vi "Write Editable From.vi"(8 "error in (no error)":errorcluster, 10 "RowAndCollumn":T1, 11 "MCListbox View in":refnum<class "MCListbox View.lvclass">) -> (0 "error out":errorcluster, 3 "MCListbox View out":refnum<class "MCListbox View.lvclass">)   [LabVIEW 2013, in "SET Project Editor.lvlib" / "MCListbox View.lvclass"]
uses:
  MCListbox View.lvclass
  <vilib>/Utility/miscctls.llb/LVRowAndColumnTypeDef.ctl
  MCListbox View.lvclass/MCListbox View.ctl
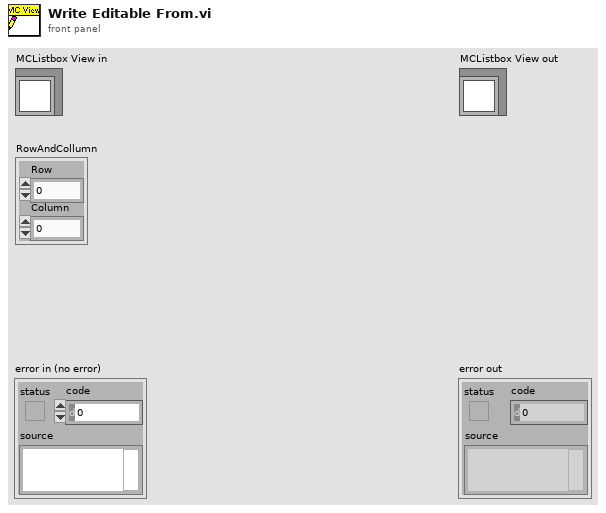
[diagram p1: front panel]
types:
  T1 = typedef "LVRowAndColumnTypeDef.ctl" = cluster{"Row":i32, "Column":i32}
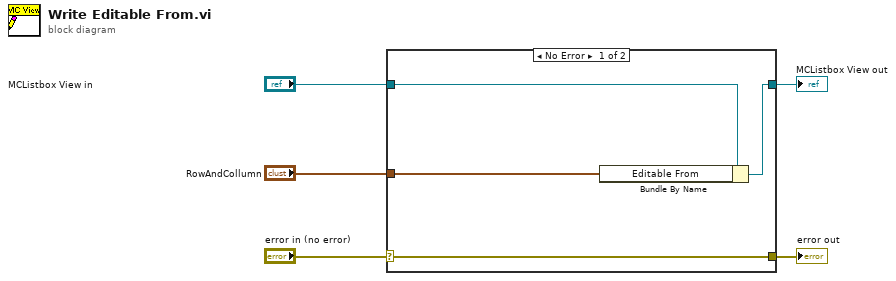
[diagram p0: block diagram]
diagram:
  n1 = case shown="No Error" "error in (no error)" {
    selector: "error in (no error)" -> [w9 w10]
    tunnel: [w9 w10] -> w4
    tunnel: [w7 w11] -> w2
    tunnel: "MCListbox View in" -> [w8 w11]
    tunnel: "RowAndCollumn" -> [w6 _]
    frame No Error {
      n2 = Bundle By Name(cluster=w8, "Editable From"=w6) -> (w7:refnum<class "MCListbox View.lvclass">)
    }
    frame Error {
    }
  }
  "error out" <- w4
  "MCListbox View out" <- w2
